vi "IsROIChange.vi"(9 "InputData":u32[](array[numeric]), 11 "ROI":T1) -> (1 "OutputData":u32[](array[numeric]), 3 "Change?":bool)   [LabVIEW 2015]
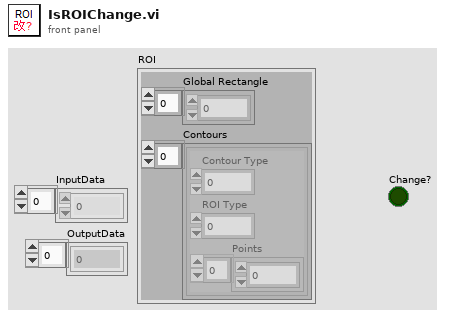
[diagram p1: front panel]
types:
  T1 = cluster{"Global Rectangle":i32[], "Contours":cluster{"Contour Type":u32, "ROI Type":u32, "Points":i32[]}[]}
  T2 = cluster{"Contour Type":u32, "ROI Type":u32, "Points":i32[]}[]
  T3 = cluster{"Contour Type":u32, "ROI Type":u32, "Points":i32[]}
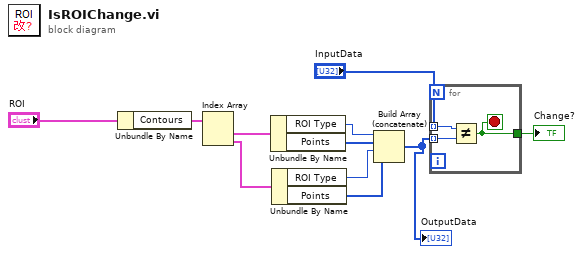
[diagram p0: block diagram]
diagram:
  n1 = Unbundle By Name("ROI") -> ("Contours"=w10:T2)
  n2 = Index Array(array=w10) -> (element #1=w11:T3, element #2=w3:T3)  [unwired: 2 in]
  n3 = Unbundle By Name(w11) -> ("ROI Type"=w9:u32, "Points"=w8:i32[])
  n4 = Unbundle By Name(w3) -> ("ROI Type"=w2:u32, "Points"=w1:i32[])
  n5 = Build Array (concatenate)(w9, w8, w2, w1) -> (w4:u32[])
  "OutputData" <- w4
  n6 = for {
    tunnel: "InputData" -> [w14] mode=indexing
    tunnel: w4 -> [w13] mode=indexing
    tunnel: [w12] -> w6
    stop <- w12 stop-if-true
    n7 = Not Equal?(x=w14, y=w13) -> (x != y?=w12:bool)
  }
  "Change?" <- w6
